vi "draw_Cernox_R2T.vi"() -> ()   [LabVIEW 2019]
panel:
  in  "Cernox ID":enum16{"X130217"}(ring)
  out "XY Graph":cluster{dbl[], dbl[]}(graph)
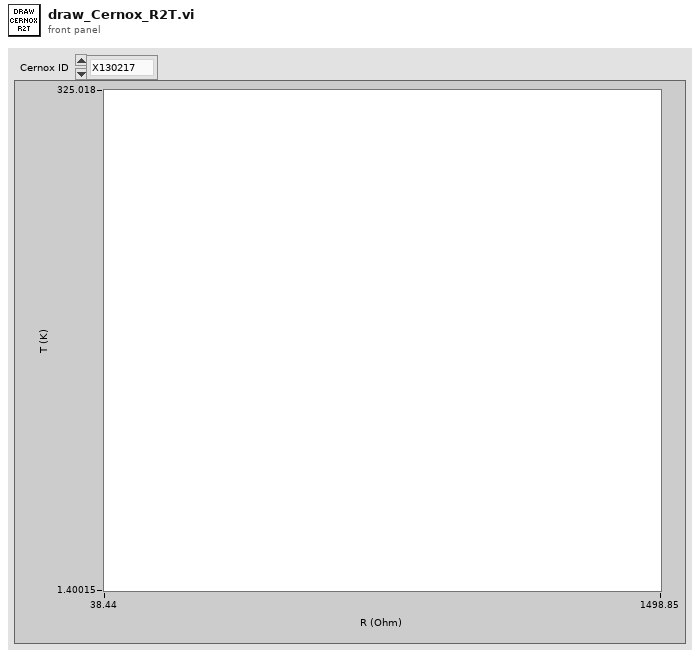
[diagram p1: front panel]
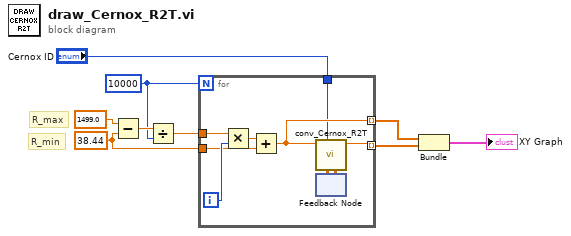
[diagram p0: block diagram]
diagram:
  w2 = 38.44
  w4 = 10000
  # "R_max"
  # "R_min"
  n1 = Subtract(x=1499.0, y=w2) -> (x-y=w5:dbl)
  n2 = Divide(x=w5, y=w4) -> (x/y=w3:dbl)
  n3 = for {
    N: w4 -> [_]
    tunnel: w3 -> [w18]
    tunnel: w2 -> [w15]
    tunnel: [w11] -> w9 mode=indexing
    tunnel: [w12] -> w8 mode=indexing
    tunnel: "Cernox ID" -> [w10]
    i -> [w17]
    n4 = Multiply(x=w18, y=w17) -> (x*y=w16:dbl)
    n5 = Add(x=w16, y=w15) -> (x+y=w11:dbl)
    n6 = feedback #1() -> (w13:dbl[][])  [unwired: 1 in]
    n7 = call "conv_Cernox_R2T.vi"("data_in"=w13, "Cernox ID"=w10, "R"=w11) -> ("T"=w12:dbl, "data_out"=w14:dbl[][])  [unwired: 6 in, 1 out]
    n8 = feedback-in #1(w14) -> ()
  }
  n9 = Bundle(w9, w8) -> (→"XY Graph":cluster{dbl[], dbl[]})  [unwired: 1 in]
